vi "Check Settings.vi"(8 "error in (no error)":errorcluster, 10 "Iterator Settings":T1={"Prepare timeout (ms)"=200, "Iterate timeout (ms)"=50, "Conclude timeout (ms)"=200, "Iterate period (ms)"=200, "Number of iterations"=5, "Time before stop (ms)"=5, "Active Stop Conditions"={"Number of Iterations"=FALSE, "Time Elapsed"=FALSE, "Iteration Result"=FALSE}, "Prepare Msg"=refnum, "Iterate Msg"=refnum, "Conclude Msg"=refnum, "Iterations End Report"=refnum, "Message Priority (Normal)"=enum."Normal"}, 11 "Iterator NR Actor in":refnum<class "Iterator NR Actor.lvclass">) -> (0 "error out":errorcluster, 2 "Iterator Settings out":T1={"Prepare timeout (ms)"=200, "Iterate timeout (ms)"=50, "Conclude timeout (ms)"=200, "Iterate period (ms)"=200, "Number of iterations"=5, "Time before stop (ms)"=5, "Active Stop Conditions"={"Number of Iterations"=FALSE, "Time Elapsed"=FALSE, "Iteration Result"=FALSE}, "Prepare Msg"=refnum, "Iterate Msg"=refnum, "Conclude Msg"=refnum, "Iterations End Report"=refnum, "Message Priority (Normal)"=enum."Normal"}, 3 "Iterator NR Actor out":refnum<class "Iterator NR Actor.lvclass">)   [LabVIEW 2023, in "Iterator Actor.lvlib" / "Iterator NR Actor.lvclass"]
doc: "Checks the input settings of the iterator. \nReturns an error with a description if something is wrong."
uses:
  Iterator NR Actor.lvclass
  Abstract Iterator Actor/Iterator Settings.ctl
  Abstract Iterator Actor Messages/Iterator Report Iterations End Msg/Iterator Report Iterations End Msg.lvclass
  <vilib>/ActorFramework/Message/Message.lvclass
  Abstract Iterator Actor/Active Stop Conditions.ctl
  <vilib>/ActorFramework/Message Enqueuer/Message Priority.ctl
  <vilib>/ActorFramework/Actor/Actor.lvclass/Actor.ctl
  <vilib>/ActorFramework/Message Enqueuer/Message Enqueuer.lvclass/Message Enqueuer.ctl
  <vilib>/ActorFramework/Message Enqueuer/Init from Existing Queue.vi
  <vilib>/Utility/error.llb/Error Cluster From Error Code.vi
  Abstract Iterator Actor/Abstract Iterator Actor.lvclass
  <vilib>/ActorFramework/Message Enqueuer/Message Enqueuer.lvclass
  <vilib>/ErrorRing/Error Ring.xnode
  Iterator NR Actor.lvclass/Iterator NR Actor.ctl
  <vilib>/ActorFramework/Actor/Actor.lvclass
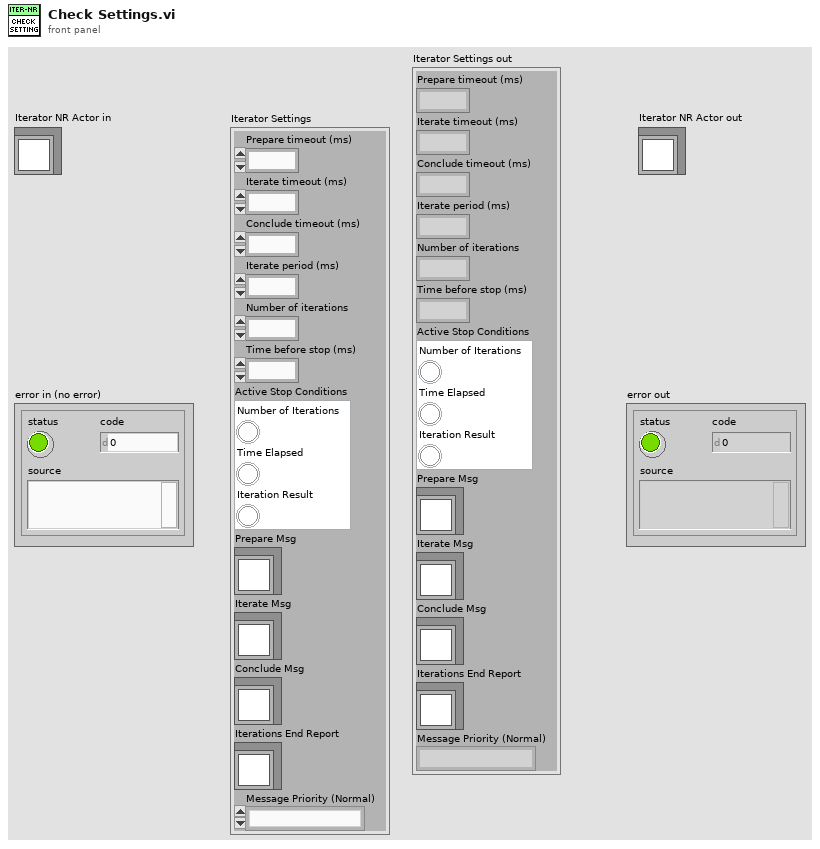
[diagram p1: front panel]
types:
  T1 = typedef "Iterator Actor.lvlib/Abstract Iterator Actor.lvclass/Iterator Settings.ctl" = cluster{"Prepare timeout (ms)":i32, "Iterate timeout (ms)":i32, "Conclude timeout (ms)":i32, "Iterate period (ms)":i32, "Number of iterations":i32, "Time before stop (ms)":i32, "Active Stop Conditions":T2, "Prepare Msg":refnum<class "Message.lvclass">, "Iterate Msg":refnum<class "Message.lvclass">, "Conclude Msg":refnum<class "Message.lvclass">, "Iterations End Report":refnum<class "Iterator Report Iterations End Msg.lvclass">, "Message Priority (Normal)":T3}
  T2 = typedef "Iterator Actor.lvlib/Abstract Iterator Actor.lvclass/Active Stop Conditions.ctl" = cluster{"Number of Iterations":bool, "Time Elapsed":bool, "Iteration Result":bool}
  T3 = typedef "Actor Framework.lvlib/Message Enqueuer.lvclass/Message Priority.ctl" = enum16{"Low", "Normal", "High"}
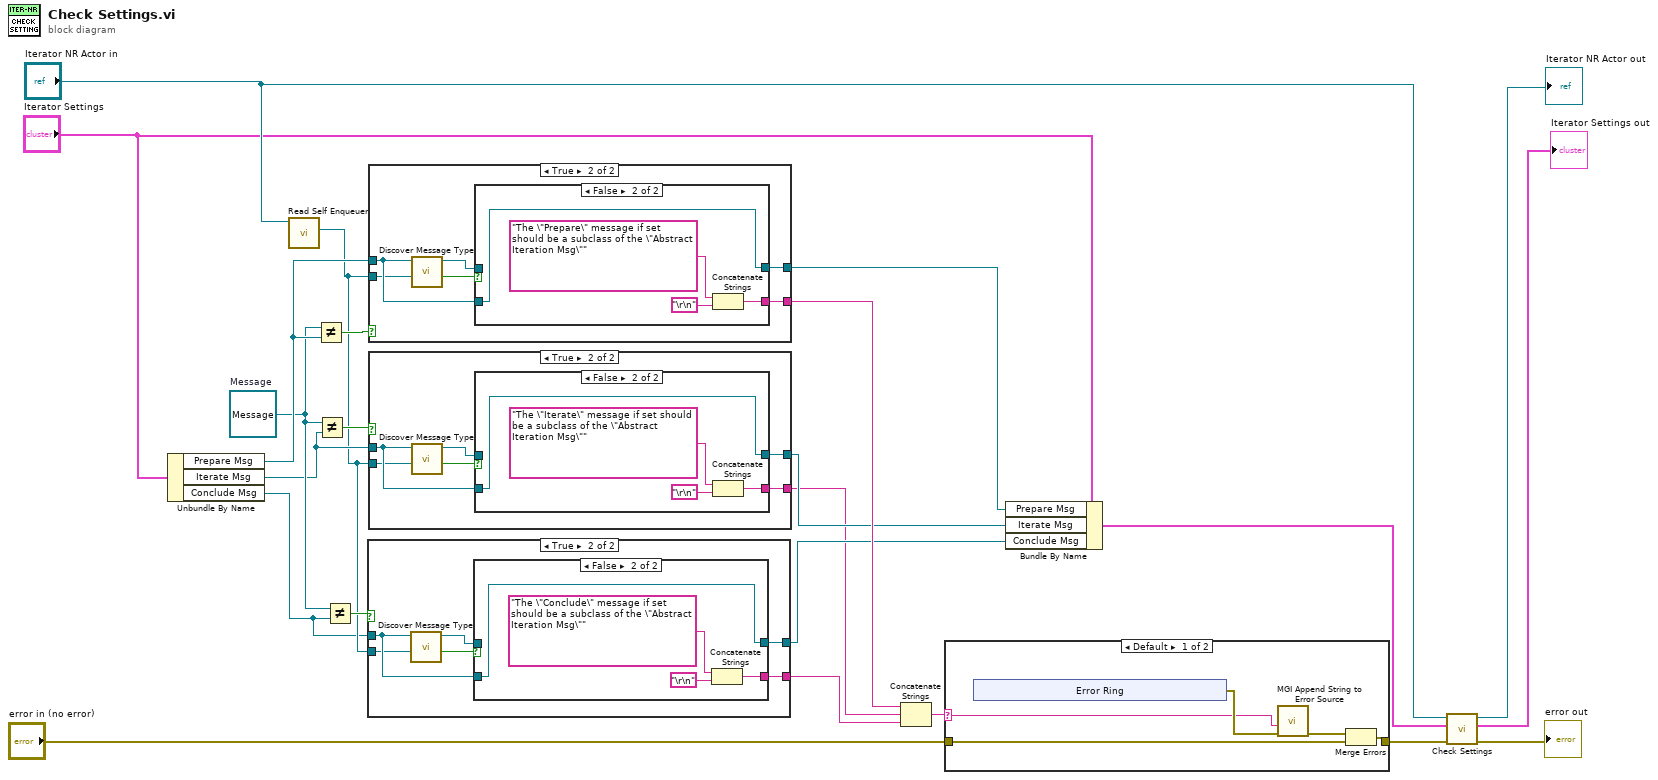
[diagram p0: block diagram]
diagram:
  w21 = refnum<class "Message.lvclass"> refnum  # Message
  n1 = Unbundle By Name("Iterator Settings") -> ("Prepare Msg"=w22:refnum<class "Message.lvclass">, "Iterate Msg"=w8:refnum<class "Message.lvclass">, "Conclude Msg"=w5:refnum<class "Message.lvclass">)
  n2 = call <vilib>:"Read Self Enqueuer.vi"("Actor"="Iterator NR Actor in") -> ("Self Enqueuer"=w6:refnum<class "Message Enqueuer.lvclass">)  [unwired: 10 in]
  n3 = Not Equal?(x=w21, y=w22) -> (x != y?=w23:bool)
  n4 = Not Equal?(x=w21, y=w8) -> (x != y?=w9:bool)
  n5 = Not Equal?(x=w21, y=w5) -> (x != y?=w7:bool)
  n6 = case shown="True" w7 {
    tunnel: w5 -> [w24 w27]
    tunnel: [_ w29] -> w1
    tunnel: [w24 w26] -> w3
    tunnel: w6 -> [_ w25]
    frame False {
    }
    frame True {
      n7 = call "Discover Message Type.vi"("Message Enqueuer"=w25, "Message in"=w27) -> ("Message Valid"=w30:bool, "Message out"=w28:refnum<class "Message.lvclass">)  [unwired: 8 in]
      n8 = case shown="False" w30 {
        tunnel: [_ w33] -> w29
        tunnel: w28 -> [w31 _]
        tunnel: [w31 w32] -> w26
        tunnel: w27 -> [_ w32]
        frame True {
        }
        frame False {
          n9 = Concatenate Strings("The \"Conclude\" message if set should be a subclass of the \"Abstract Iteration Msg\"", "\r\n") -> (w33:string)
        }
      }
    }
  }
  n10 = case shown="True" w23 {
    tunnel: w22 -> [w36 w39]
    tunnel: [_ w41] -> w20
    tunnel: [w36 w38] -> w14
    tunnel: w6 -> [_ w37]
    frame False {
    }
    frame True {
      n11 = call "Discover Message Type.vi"("Message Enqueuer"=w37, "Message in"=w39) -> ("Message Valid"=w42:bool, "Message out"=w40:refnum<class "Message.lvclass">)  [unwired: 8 in]
      n12 = case shown="False" w42 {
        tunnel: [_ w45] -> w41
        tunnel: w40 -> [w43 _]
        tunnel: [w43 w44] -> w38
        tunnel: w39 -> [_ w44]
        frame True {
        }
        frame False {
          n13 = Concatenate Strings("The \"Prepare\" message if set should be a subclass of the \"Abstract Iteration Msg\"", "\r\n") -> (w45:string)
        }
      }
    }
  }
  n14 = case shown="True" w9 {
    tunnel: w8 -> [w48 w51]
    tunnel: [_ w53] -> w2
    tunnel: [w48 w50] -> w4
    tunnel: w6 -> [_ w49]
    frame False {
    }
    frame True {
      n15 = call "Discover Message Type.vi"("Message Enqueuer"=w49, "Message in"=w51) -> ("Message Valid"=w54:bool, "Message out"=w52:refnum<class "Message.lvclass">)  [unwired: 8 in]
      n16 = case shown="False" w54 {
        tunnel: [_ w57] -> w53
        tunnel: w52 -> [w55 _]
        tunnel: [w55 w56] -> w50
        tunnel: w51 -> [_ w56]
        frame True {
        }
        frame False {
          n17 = Concatenate Strings("The \"Iterate\" message if set should be a subclass of the \"Abstract Iteration Msg\"", "\r\n") -> (w57:string)
        }
      }
    }
  }
  n18 = Concatenate Strings(w20, w2, w1) -> (w19:string)
  n19 = case shown="Default" w19 {
    selector: w19 -> [w60 _]
    tunnel: "error in (no error)" -> [w64 w69]
    tunnel: [w63 w69] -> w18
    frame Default {
      n20 = xnode "Error Ring"() -> ("error out"=w62:errorcluster)
      n21 = call <userlib>:"MGI Append String to Error Source.vi"("Error In"=w62, "String to Append"=w60) -> ("Error Out"=w61:errorcluster)  [unwired: 9 in]
      n22 = Merge Errors(w61, w64) -> (w63:errorcluster)
    }
    frame "" {
    }
  }
  n23 = Bundle By Name(cluster="Iterator Settings", "Prepare Msg"=w14, "Iterate Msg"=w4, "Conclude Msg"=w3) -> (w10:T1)
  n24 = call-parent "Check Settings.vi"("error in (no error)"=w18, "Iterator Settings in"=w10, "Abstract Iterator Actor in"="Iterator NR Actor in") -> ("error out"=→"error out":errorcluster, "Iterator Settings out"=→"Iterator Settings out":T1, "Abstract Iterator Actor out"=→"Iterator NR Actor out":refnum<class "Iterator NR Actor.lvclass">)  [unwired: 6 in]
